vi "Close.vi"(8 "error in (no error)":errorcluster, 11 "Data in":refnum<class "FPGA-Bus_SGL.lvclass">) -> (0 "error out":errorcluster, 3 "Data out":refnum<class "FPGA-Bus_SGL.lvclass">)   [LabVIEW 2021, in "FPGA-Bus_SGL.lvclass"]
uses:
  FPGA-Bus_SGL.lvclass
  FPGA-Bus_SGL.lvclass/FPGA-Bus_SGL.ctl
  <vilib>/FPGAPlugInAG/Dynamic/niLvFpga_Close_Dynamic.vi
  <vilib>/rvi/interface/nirviCloseFPGA/nirviCloseFPGA.xnode
  Support/FPGA Type.ctl
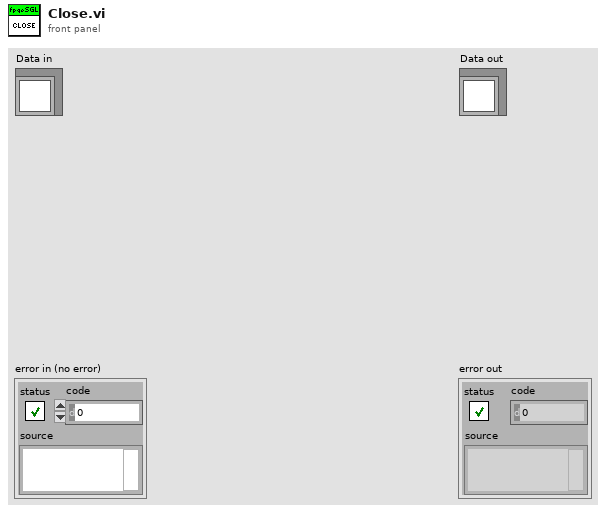
[diagram p1: front panel]
types:
  T1 = typedef "FPGA-Bus_SGL.lvclass/FPGA Type.ctl" = refnum<k20>
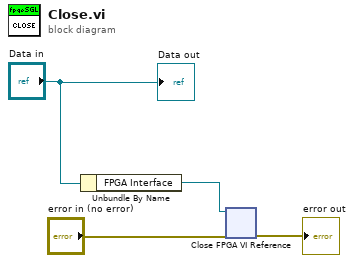
[diagram p0: block diagram]
diagram:
  n1 = Unbundle By Name("Data in") -> ("FPGA Interface"=w1:T1)
  n2 = xnode "Close FPGA VI Reference"("FPGA VI Reference In"=w1, "error in"="error in (no error)") -> ("error out"=→"error out":errorcluster)
  "Data out" <- "Data in"
